vi "MotorCommunication.vi"(5 "Question":string, 6 "error out":errorcluster caption="error in", 9 "COM Port in":refnum<visa-resource-name>) -> (0 "error IO":errorcluster caption="error out", 3 "COM Port out":refnum<visa-resource-name>, 4 "Answer":string)   [LabVIEW 2009]
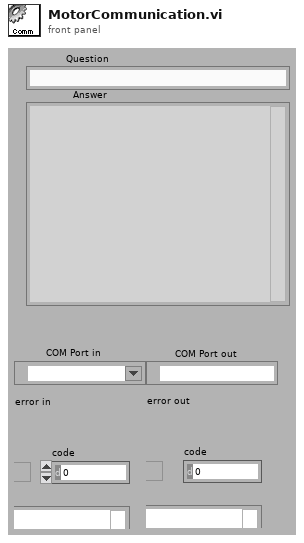
[diagram p1: front panel]
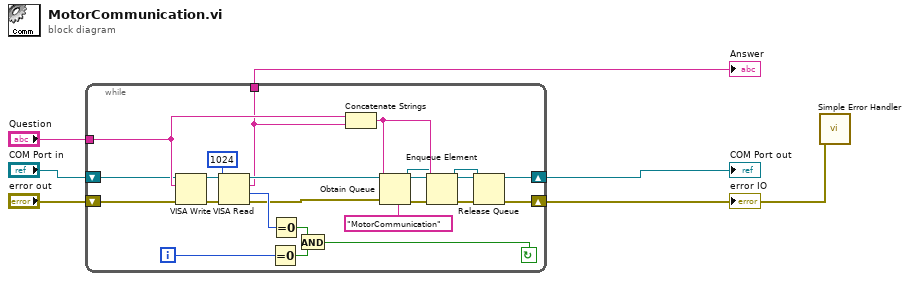
[diagram p0: block diagram]
diagram:
  n1 = while {
    tunnel: "Question" -> [w12]
    shift-right: [w11] -> w3
    shift-left: "error out" -> [w8]
    tunnel: [w10] -> w2
    shift-right: [w27] -> w1
    shift-left: "COM Port in" -> [w9]
    i -> [w22]
    stop <- w19 continue-if-true
    n2 = VISA Write(VISA resource name=w9, write buffer=w12, error in (no error)=w8) -> (VISA resource name out=w24:refnum<visa-resource-name>, error out=w25:errorcluster)  [unwired: 1 out]
    n3 = VISA Read(VISA resource name=w24, byte count=u32 1024 ("nombre d'octets (0)"), error in (no error)=w25) -> (VISA resource name out=w27:refnum<visa-resource-name>, read buffer=w10:string, return count=w23:u32, error out=w7:errorcluster)
    n4 = Equal To 0?(x=w22) -> (x = 0?=w20:bool)
    n5 = Equal To 0?(x=w23) -> (x = 0?=w21:bool)
    n6 = And(x=w21, y=w20) -> (x .and. y?=w19:bool)
    n7 = Concatenate Strings(w12, w10) -> (w15:string)
    n8 = Obtain Queue(name (unnamed)="MotorCommunication" ("nom (aucun)"), element data type=w15, error in (no error)=w7) -> (queue out=w14:refnum<queue>, error out=w13:errorcluster)  [unwired: 2 in, 1 out]
    n9 = Enqueue Element(queue=w14, element=w15, error in (no error)=w13) -> (queue out=w16:refnum<queue>, error out=w17:errorcluster)  [unwired: 2 out]
    n10 = Release Queue(queue=w16, error in (no error)=w17) -> (error out=w11:errorcluster)  [unwired: 3 out]
  }
  "Answer" <- w2
  "error IO" <- w3
  "COM Port out" <- w1
  n11 = call <vilib>:"Simple Error Handler.vi"("error in (no error)"=w3) -> ()  [unwired: 1 in, 8 out]
